vi "AuMT8852B Single Payload Configuration.vi"(5 "Settings":T1={"Test control"=enum."Loopback", "Payload"=enum."10101010", "Hopping"=enum."Hopping off", "TX frequency"=2441.0, "RX frequency"=2402.0, "Use Dirty transmitter"=FALSE, "Packet type"=enum."DH1"}, 7 "Set/Get (Set)":enum16{"Set", "Get"}(ring), 8 "error in (no error)":errorcluster, 10 "Script (3)":i32=3, 11 "VISA session":refnum<visa-resource-name>) -> (0 "error out":errorcluster, 2 "error code":i32, 3 "VISA session out":refnum<visa-resource-name>, 4 "Settings out":T1={"Test control"=enum."Loopback", "Payload"=enum."10101010", "Hopping"=enum."Hopping off", "TX frequency"=2441.0, "RX frequency"=2402.0, "Use Dirty transmitter"=FALSE, "Packet type"=enum."DH1"})   [LabVIEW 2017]
doc: "Anritsu MT8852B Bluetooth Tester\n\nConfigures how Carrier, Sensitivity, and other tests are carried out when script mode is set to Single Payload. Note that the Maximum Input Power Sensitivity Test is not supported in Single Payload mode.\n\nINPUTS\nSet/Get - whether the values are being sent to or retrieved from the instrument.\nScript - which of the stored scripts (1-10) will be queried or configured. Scripts 1 and 2 are read-only.\nSettings - parameters of the single payload mode to be written.\n\nOUTPUTS\nSettings out - current parameters of the single payload mode."
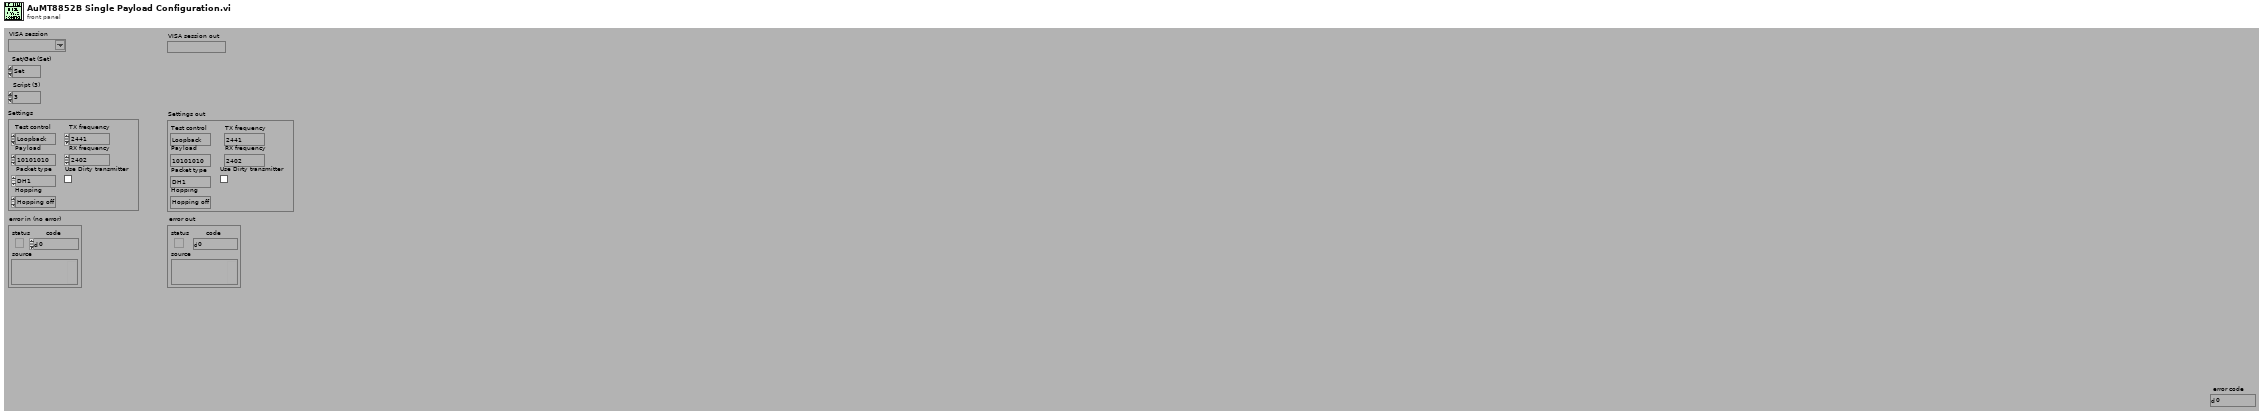
[diagram p1: front panel]
types:
  T1 = cluster{"Test control":enum16{"Loopback", "TX test"}, "Payload":enum16{"10101010", "11110000", "PRBS-9"}, "Hopping":enum16{"Hopping off", "Hopping on"}, "TX frequency":dbl, "RX frequency":dbl, "Use Dirty transmitter":bool, "Packet type":enum16{"DH1", "DH3", "DH5", "2-DH1", "2-DH3", "2-DH5", "3-DH1", "3-DH3", "3-DH5"}}
  T2 = enum16{"DH1", "DH3", "DH5", "2-DH1", "2-DH3", "2-DH5", "3-DH1", "3-DH3", "3-DH5"}
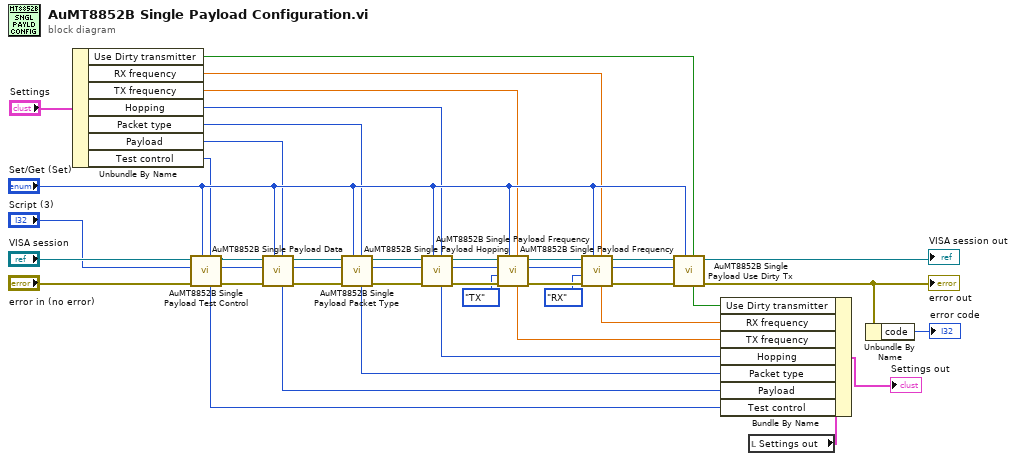
[diagram p0: block diagram]
diagram:
  n1 = Unbundle By Name("Settings") -> ("Use Dirty transmitter"=w15:bool, "RX frequency"=w16:dbl, "TX frequency"=w17:dbl, "Hopping"=w18:enum16{"Hopping off", "Hopping on"}, "Packet type"=w19:T2, "Payload"=w20:enum16{"10101010", "11110000", "PRBS-9"}, "Test control"=w21:enum16{"Loopback", "TX test"})
  n2 = call <instrlib>:"AuMT8852B Single Payload Test Control.vi"("Test control (Loopback)"=w21, "Set/Get (Set)"="Set/Get (Set)", "error in (no error)"="error in (no error)", "Script (3)"="Script (3)", "VISA session"="VISA session") -> ("error out"=w34:errorcluster, "VISA session out"=w35:refnum<visa-resource-name>, "Test control out"=w9:enum16{"Loopback", "TX test"})  [unwired: 3 in, 1 out]
  n3 = call <instrlib>:"AuMT8852B Single Payload Data.vi"("Payload (10101010)"=w20, "Set/Get (Set)"="Set/Get (Set)", "error in (no error)"=w34, "Script (3)"="Script (3)", "VISA session"=w35) -> ("error out"=w25:errorcluster, "VISA session out"=w24:refnum<visa-resource-name>, "Payload out"=w10:enum16{"10101010", "11110000", "PRBS-9"})  [unwired: 3 in, 1 out]
  n4 = call <instrlib>:"AuMT8852B Single Payload Packet Type.vi"("Packet type (DH5)"=w19, "Set/Get (Set)"="Set/Get (Set)", "error in (no error)"=w25, "Script (3)"="Script (3)", "VISA session"=w24) -> ("error out"=w22:errorcluster, "VISA session out"=w23:refnum<visa-resource-name>, "Packet type out"=w2:T2)  [unwired: 3 in, 1 out]
  n5 = call <instrlib>:"AuMT8852B Single Payload Hopping.vi"("Hopping (Hopping off)"=w18, "Set/Get (Set)"="Set/Get (Set)", "error in (no error)"=w22, "Script (3)"="Script (3)", "VISA session"=w23) -> ("error out"=w33:errorcluster, "VISA session out"=w32:refnum<visa-resource-name>, "Hopping out"=w11:enum16{"Hopping off", "Hopping on"})  [unwired: 3 in, 1 out]
  n6 = call <instrlib>:"AuMT8852B Single Payload Frequency.vi"("Frequency (2441 MHz)"=w17, "Set/Get (Set)"="Set/Get (Set)", "error in (no error)"=w33, "Type (TX)"=enum16{"TX", "RX"}."TX", "Script (3)"="Script (3)", "VISA session"=w32) -> ("error out"=w31:errorcluster, "VISA session out"=w30:refnum<visa-resource-name>, "Frequency out"=w12:dbl)  [unwired: 2 in, 1 out]
  n7 = call <instrlib>:"AuMT8852B Single Payload Frequency.vi"("Frequency (2441 MHz)"=w16, "Set/Get (Set)"="Set/Get (Set)", "error in (no error)"=w31, "Type (TX)"=enum16{"TX", "RX"}."RX", "Script (3)"="Script (3)", "VISA session"=w30) -> ("error out"=w29:errorcluster, "VISA session out"=w28:refnum<visa-resource-name>, "Frequency out"=w13:dbl)  [unwired: 2 in, 1 out]
  n8 = call <instrlib>:"AuMT8852B Single Payload Use Dirty Tx.vi"("Use Dirty transmitter? (F)"=w15, "Set/Get (Set)"="Set/Get (Set)", "error in (no error)"=w29, "Script (3)"="Script (3)", "VISA session"=w28) -> ("error out"=w7:errorcluster, "VISA session out"=→"VISA session out":refnum<visa-resource-name>, "Use Dirty transmitter? out"=w14:bool)  [unwired: 3 in, 1 out]
  "error out" <- w7
  n9 = local read "Settings out"() -> (w3:T1)
  n10 = Bundle By Name(cluster=w3, "Use Dirty transmitter"=w14, "RX frequency"=w13, "TX frequency"=w12, "Hopping"=w11, "Packet type"=w2, "Payload"=w10, "Test control"=w9) -> (→"Settings out":T1)
  n11 = Unbundle By Name(w7) -> ("code"=→"error code":i32)
